vi "Read data.vi"(8 "error in (no error)":errorcluster, 10 "Buffer mode":T1, 11 "Scope5761 in":refnum<class "Scope5761.lvclass">) -> (0 "error out":errorcluster, 1 "Any read?":bool, 2 "Data":dbl[][](array[numeric]), 3 "Scope5761 out":refnum<class "Scope5761.lvclass">)   [LabVIEW 2013, in "Scope5761.lvclass"]
uses:
  Scope5761.lvclass
  ScopeBase/ScopeBase.lvclass
  controls/Data_display_mode.ctl
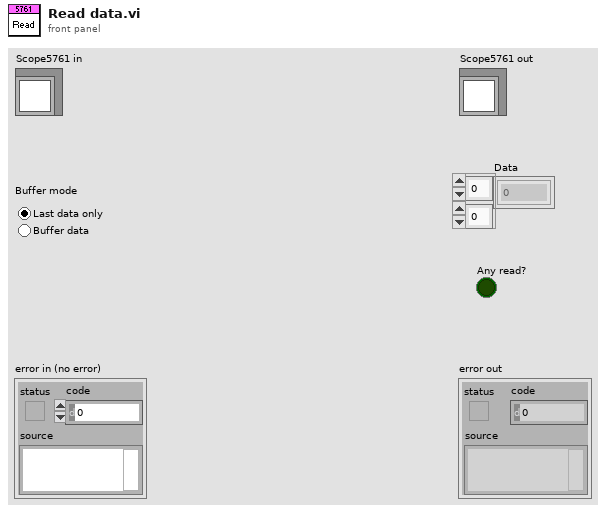
[diagram p1: front panel]
types:
  T1 = typedef "Data_display_mode.ctl" = enum32{"Last data only", "Buffer data"}
  T2 = typedef "ScopeMode.ctl" = enum16{"Stopped", "Single", "Running", "Continuous"}
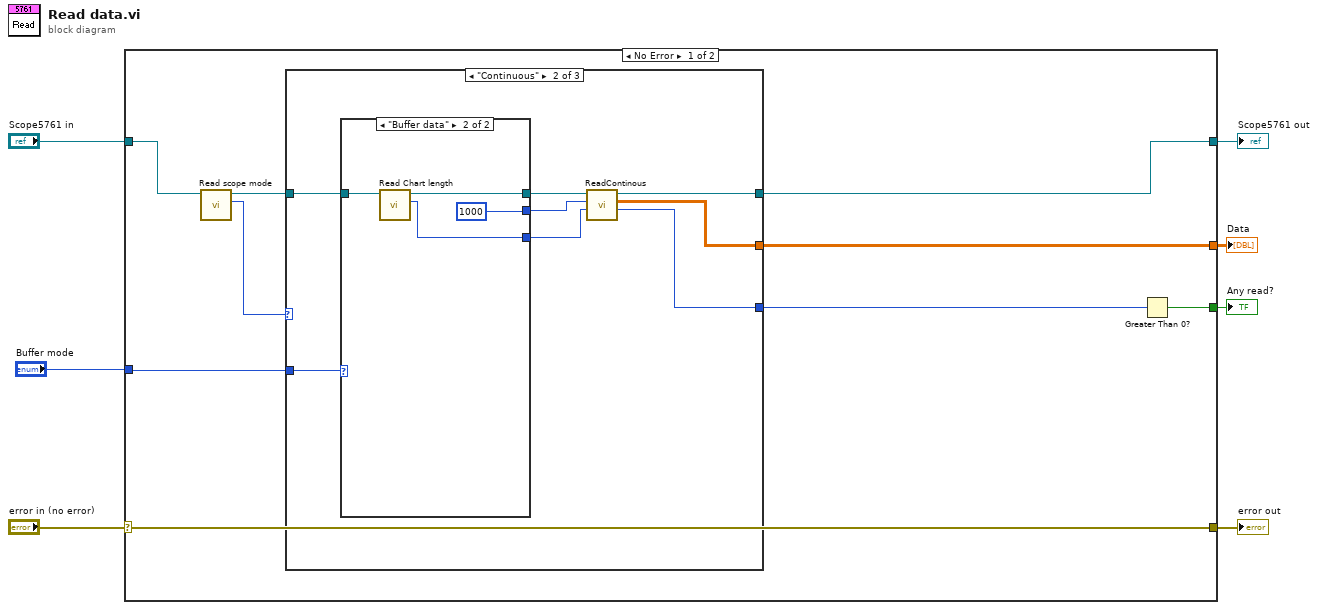
[diagram p0: block diagram]
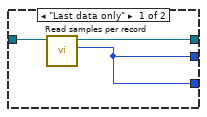
[diagram p3: hidden frame]
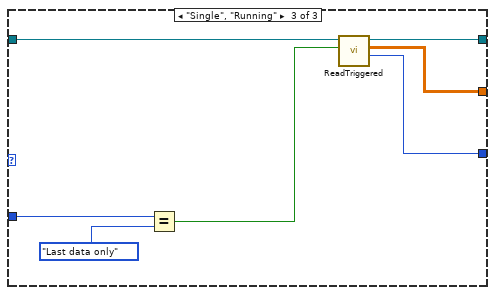
[diagram p4: hidden frame]
diagram:
  n1 = case shown="No Error" "error in (no error)" {
    selector: "error in (no error)" -> [w16 w41]
    tunnel: [w16 w41] -> w6
    tunnel: [w12 w40] -> w4
    tunnel: "Scope5761 in" -> [w15 w40]
    tunnel: "Buffer mode" -> [w8 _]
    tunnel: [w11 _] -> w1
    tunnel: [w9 _] -> w2
    frame No Error {
      n2 = call "Read scope mode.vi"("ScopeBase in"=w15) -> ("scope mode"=w13:T2, "ScopeBase out"=w14:refnum<class "Scope5761.lvclass">)  [unwired: 8 in, 1 out]
      n3 = case shown="\"Continuous\"" w13 {
        tunnel: w14 -> [w17 w19 w39]
        tunnel: [w17 w25 w38] -> w12
        tunnel: [_ w24 w37] -> w11
        tunnel: [_ w23 w36] -> w10
        tunnel: w8 -> [_ w22 w34]
        frame "Stopped", Default {
        }
        frame "Continuous" {
          n4 = case shown="\"Buffer data\"" w22 {
            tunnel: [w27 1000 ("Min samples to read")] -> w21
            tunnel: [w27 w30] -> w20
            tunnel: w19 -> [w28 w32]
            tunnel: [w26 w31] -> w18
            frame "Last data only" {
              n5 = call "Read samples per record.vi"("ScopeBase in"=w28) -> ("samples per record"=w27:i32, "ScopeBase out"=w26:refnum<class "Scope5761.lvclass">)  [unwired: 8 in, 1 out]
            }
            frame "Buffer data" {
              n6 = call "Read Chart length.vi"("ScopeBase in"=w32) -> ("Chart length"=w30:i32, "ScopeBase out"=w31:refnum<class "Scope5761.lvclass">)  [unwired: 8 in, 1 out]
            }
          }
          n7 = call-dynamic "ReadContinous.vi"("Max samples to keep"=w20, "Min samples to read"=w21, "Scope5761 in"=w18) -> ("#elements"=w23:i32, "Data"=w24:dbl[][], "Scope5761 out"=w25:refnum<class "Scope5761.lvclass">)  [unwired: 5 in, 1 out]
        }
        frame "Single", "Running" {
          n8 = Equal?(x=w34, y=Data_display_mode."Last data only") -> (x = y?=w33:bool)
          n9 = call-dynamic "ReadTriggered.vi"("Keep last record only"=w33, "Scope5761 in"=w39) -> ("#elements"=w36:i32, "Data"=w37:dbl[][], "Scope5761 out"=w38:refnum<class "Scope5761.lvclass">)  [unwired: 6 in, 1 out]
        }
      }
      n10 = Greater Than 0?(x=w10) -> (x > 0?=w9:bool)
    }
    frame Error {
    }
  }
  "error out" <- w6
  "Scope5761 out" <- w4
  "Any read?" <- w2
  "Data" <- w1
